vi "Write log.vi"(8 "error in (no error)":errorcluster, 10 "event data":string, 11 "event":string) -> (0 "error out":errorcluster)   [LabVIEW 2015]
doc: "Write data into log file."
uses:
  <vilib>/Utility/file.llb/Write Delimited Spreadsheet (string).vi
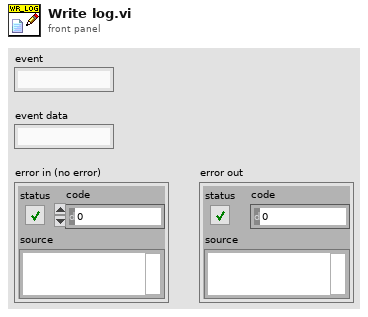
[diagram p1: front panel]
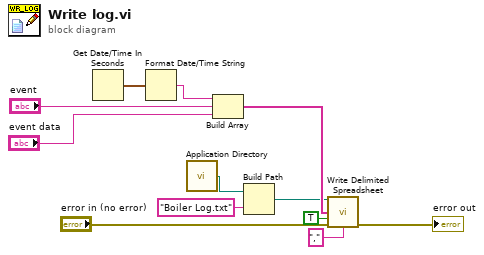
[diagram p0: block diagram]
diagram:
  n1 = Get Date/Time In Seconds() -> (seconds since 1Jan1904=w6:timestamp)
  n2 = Format Date/Time String(seconds (now)=w6) -> (date/time string=w7:string)  [unwired: 2 in]
  n3 = call <vilib>:"Application Directory.vi"() -> ("Application Directory"=w1:path)
  n4 = Build Array(w7, "event", "event data") -> (w10:string[])
  n5 = Build Path(base path=w1, name or relative path="Boiler Log.txt") -> (appended path=w3:path)
  n6 = call-poly <vilib>:"Write Delimited Spreadsheet.vi"("file path (dialog if empty)"=w3, "1D data"=w10, "append to file? (F)"=TRUE, "error in (no error)"="error in (no error)", "delimiter (\\t)"="," ("delimiter (\\t)")) -> ("error out"=→"error out":errorcluster)  [unwired: 9 in, 1 out]
